vi "Panel Power Setting.vi"() -> (6 "Dryer Type Out":string(combo), 8 "Chroma Power Setting Out":string)   [LabVIEW 2012]
uses:
  Global Test Variables DPT.vi
panel:
  in  "Dryer Type":string(combo)
  in  "Chroma Power Setting":string(combo)
  in  "stop":bool
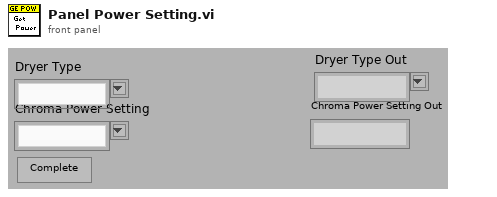
[diagram p1: front panel]
types:
  T1 = typedef "DPT Global Type.ctl" = cluster{"Test Setup":cluster{"RH Resistor":dbl, "Temp Cal":dbl, "Temp Coeff":dbl, "Power On Threshold":dbl, "MA Filter Size":i32, "Weight Offset":dbl, "Temp Resistor":dbl, "Gas Enabled":bool, "Gas P. Resistor":dbl, "Scale Com":dbl, "W. Samps":i32, "Temp4mA Val":dbl, "Temp20mA Val":dbl, "RH4mA Val":dbl, "RH20mA Val":dbl, "GPres4mA Val":dbl, "Gpres20mA Val":dbl, "Smoothing":bool, "CDAQ":bool, "34970":bool, "34980":bool, "RH-IP":string, "RH-IP2":string, "RH-IP3":string, "CompVolume":dbl, "T45_Coeff.":dbl}, "Agilent Setup":cluster{"Scale Channel":string, "TC Channels":string, "VDC Discrete Channels":string, "RH Chan":string, "Temp Chan":string, "Tscale Channel":string, "RDB Channel":string, "Gas Temperature":string, "Gas Pressure":string, "Barometric Pressure":string, "Gas Feedback Chan":string}, "Directories":cluster{"Work File Directory":path, "Save File Directory":path, "Library Directory":path, "Data Backup Directory":path, "Data Backup Dir Fail":path, "Lab Directory":path}, "Test Information":cluster{"Model:":string, "Temperature:":string, "Engineer:":string, "Technician:":string, "Comments:":string, "Lab ID:":string, "TR Number:":string, "Test Number:":string, "Test Station:":string, "Empty Dryer Cold Weight:":dbl, "Serial Number:":string, "Build:":string, "Dryer Type":string, "Humidity":string, "Test Title per TR:":string}, "cDAQ Array Locations":cluster{"Scale Channel":string, "TC Channels":string, "VDC Discrete Channel":string, "RH Chan":string, "Temp Chan":string, "Tscale Channel":string, "RDB Channel":string, "Gas Temperature":string, "Gas Pressure":string, "Barometric Pressure":string, "Gas Feedback Chan":string}}
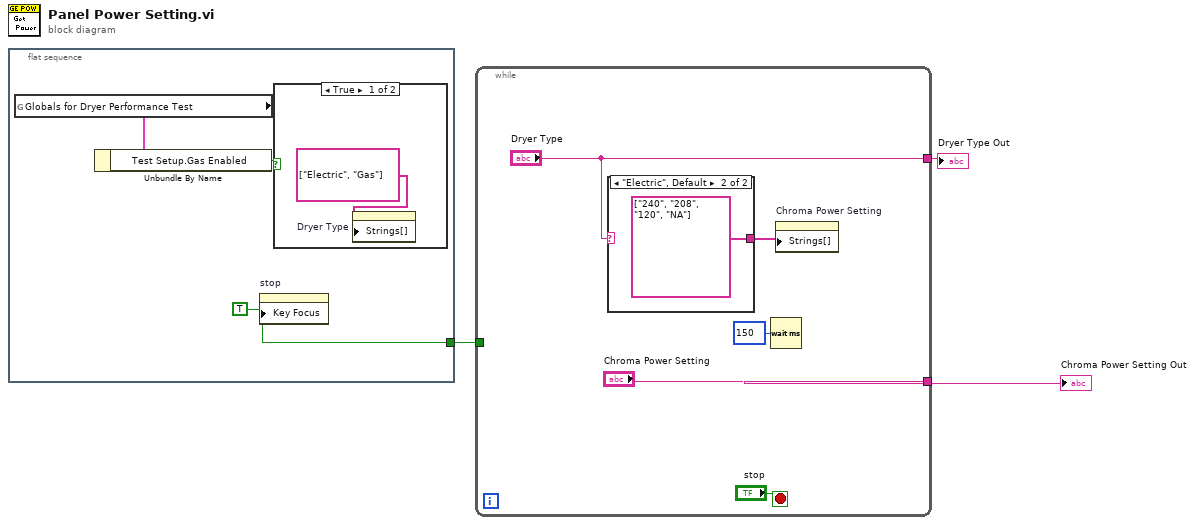
[diagram p0: block diagram]
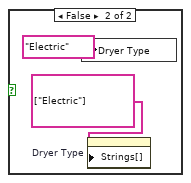
[diagram p2: hidden frame]
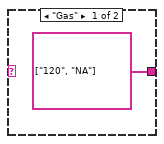
[diagram p3: hidden frame]
diagram:
  n1 = flat-sequence {
    tunnel: [w4] -> w1
    frame #0 {
      w4 = TRUE ("Key Focus")
      n2 = global read "Global Test Variables DPT.vi" "Globals for Dryer Performance Test"() -> (w6:T1)
      n3 = Unbundle By Name(w6) -> ("Test Setup.Gas Enabled"=w5:bool)
      n4 = property on="stop" class="Bool"("Key Focus"=w4) -> ()  [unwired: 2 in, 2 out]
      n5 = case shown="True" w5 {
        frame True {
          n6 = property on="Dryer Type" class="CmbBox"("Strings[]"=string[] ["Electric", "Gas"] ("Strings [] 2")) -> ()  [unwired: 2 in, 2 out]
        }
        frame False {
          n7 = local write "Dryer Type"("Electric" ("Dryer Type")) -> ()
          n8 = property on="Dryer Type" class="CmbBox"("Strings[]"=string[] ["Electric"] ("Strings [] 2")) -> ()  [unwired: 2 in, 2 out]
        }
      }
    }
  }
  n9 = while {
    tunnel: ["Chroma Power Setting"] -> w3
    tunnel: ["Dryer Type"] -> w2
    tunnel: w1 -> [_]
    stop <- "stop" stop-if-true
    n10 = case shown="\"Electric\", Default" "Dryer Type" {
      tunnel: [string[] ["120", "NA"] ("Strings []") string[] ["240", "208", "120", "NA"] ("Strings []")] -> w11
      frame "Gas" {
      }
      frame "Electric", Default {
      }
    }
    n11 = Wait (ms)(milliseconds to wait=u32 150) -> ()  [unwired: 1 out]
    n12 = property on="Chroma Power Setting" class="CmbBox"("Strings[]"=w11) -> ()  [unwired: 2 in, 2 out]
  }
  "Chroma Power Setting Out" <- w3
  "Dryer Type Out" <- w2
